vi "MessageName.vi"() -> (2 "MessageName":string)   [LabVIEW 2020, in "BoolData.lvlib"]
uses:
  BoolData.lvlib
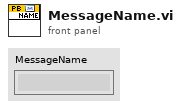
[diagram p1: front panel]
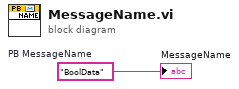
[diagram p0: block diagram]
diagram:
  w1 = "BoolData"  # PB MessageName
  "MessageName" <- w1
